vi "Read Frequencies and Voltages.vi"(0 "Function Generator.lvclass in":refnum<class "Function Generator.lvclass">, 5 "error in (no error)":errorcluster) -> (11 "array of outputs on":bool[](array[boolean]), 12 "Ch1 Frequency":dbl[unit], 13 "Ch2 Low":dbl[unit], 14 "Function Generator.lvclass out":refnum<class "Function Generator.lvclass">, 15 "Ch1 High":dbl[unit], 16 "Ch1 Low":dbl[unit], 17 "Ch2 Frequency":dbl[unit], 18 "Ch2 High":dbl[unit], 19 "error out":errorcluster)   [LabVIEW 2023, in "Function Generator.lvclass"]
uses:
  Function Generator.lvclass
  Function Generator.lvclass/Function Generator.ctl
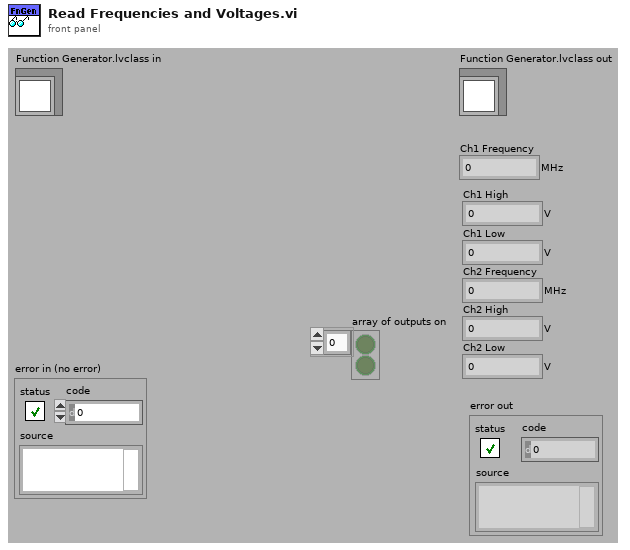
[diagram p1: front panel]
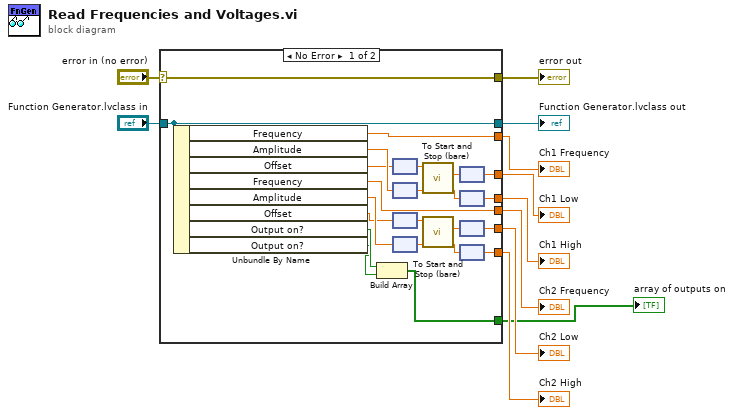
[diagram p0: block diagram]
diagram:
  n1 = case shown="No Error" "error in (no error)" {
    selector: "error in (no error)" -> [w34 w35]
    tunnel: [w34 w35] -> w10
    tunnel: [w33 w36] -> w8
    tunnel: "Function Generator.lvclass in" -> [w33 w36]
    tunnel: [w32 _] -> w7
    tunnel: [w25 _] -> w6
    tunnel: [w24 _] -> w5
    tunnel: [w23 _] -> w4
    tunnel: [w16 _] -> w3
    tunnel: [w15 _] -> w2
    tunnel: [w12 _] -> w1
    frame No Error {
      n2 = Unbundle By Name(w33) -> ("Frequency"=w32:dbl[unit], "Amplitude"=w31:dbl[unit], "Offset"=w29:dbl[unit], "Frequency"=w23:dbl[unit], "Amplitude"=w22:dbl[unit], "Offset"=w20:dbl[unit], "Output on?"=w14:bool, "Output on?"=w13:bool)
      n3 = Build Array(w14, w13) -> (w12:bool[])
      n4 = node(w29) -> (w28:dbl)
      n5 = node(w31) -> (w30:dbl)
      n6 = node(w20) -> (w19:dbl)
      n7 = node(w22) -> (w21:dbl)
      n8 = call "To Start and Stop (bare).vi"("span"=w30, "center"=w28) -> ("stop"=w26:dbl, "start"=w27:dbl)  [unwired: 4 out]
      n9 = call "To Start and Stop (bare).vi"("span"=w21, "center"=w19) -> ("stop"=w17:dbl, "start"=w18:dbl)  [unwired: 4 out]
      n10 = node(w27) -> (w24:dbl[unit])
      n11 = node(w26) -> (w25:dbl[unit])
      n12 = node(w18) -> (w15:dbl[unit])
      n13 = node(w17) -> (w16:dbl[unit])
    }
    frame Error {
    }
  }
  "error out" <- w10
  "Function Generator.lvclass out" <- w8
  "Ch1 Frequency" <- w7
  "Ch1 High" <- w6
  "Ch1 Low" <- w5
  "Ch2 Frequency" <- w4
  "Ch2 High" <- w3
  "Ch2 Low" <- w2
  "array of outputs on" <- w1
